vi "Vi 4.vi"() -> ()   [LabVIEW 2010]
panel:
  in  "stop":bool
  out "Area del triangulo":dbl(knob) scale=0.0..1000.0
  in  "Altura":dbl
  in  "Base":dbl
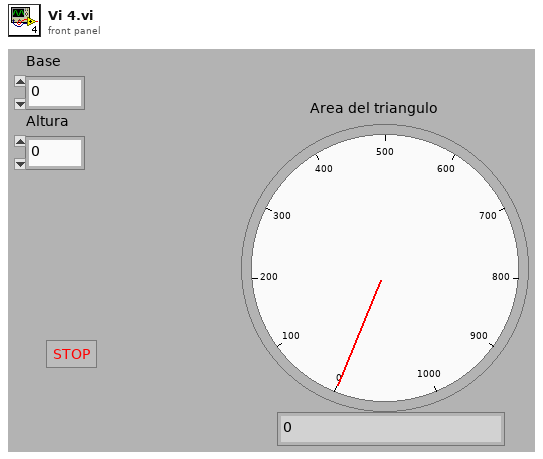
[diagram p1: front panel]
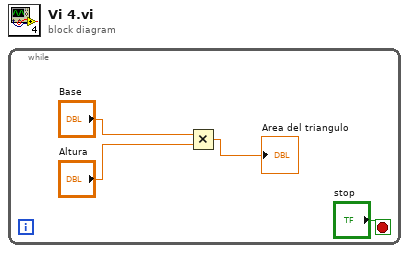
[diagram p0: block diagram]
diagram:
  n1 = while {
    stop <- "stop" stop-if-true
    n2 = Multiply(x="Base", y="Altura") -> (x*y=→"Area del triangulo":dbl)
  }
